vi "Write.vi"(6 "high priority? (F)":bool, 8 "abort (F)":bool, 9 "last element? (F)":bool, 10 "element":T2, 11 "element valid? (T)":bool=TRUE) -> (0 "done?":bool, 2 "channel":T1)   [LabVIEW 2020, in "Event Messenger Priority.lvlib"]
doc: "<p>Writes a value to an Event Messenger <a href=\"nihelplauncher://docs/csh?context=lvcore_lvconcepts_channel_wires_intro\">channel</a> so that the value can be read by one or more <a href=\"nihelplauncher://docs/csh?context=lvcore_glang_event_structure\">Event structures</a>. This endpoint waits if the channel is full.</p>"
uses:
  Event Messenger Priority.lvlib
  <vilib>/event_ctls.llb/usereventprio.ctl
  ChannelOp.ctl
  ))Channel.ctl
  Element.ctl
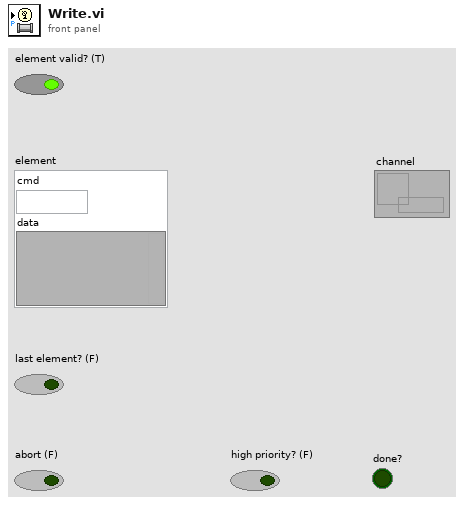
[diagram p1: front panel]
types:
  T1 = typedef "Event Messenger Priority.lvlib/))Channel.ctl" = refnum<queue>
  T2 = typedef "Event Messenger Priority.lvlib/Element.ctl" = cluster{"cmd":string, "data":variant}
  T3 = typedef "usereventprio.ctl" = enum32{"high priority", "normal priority"}
  T4 = typedef "Event Messenger Priority.lvlib/ChannelOp.ctl" = enum16{"init", "write", "register", "replicate", "probe"}
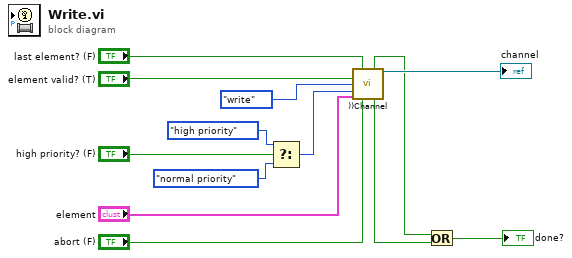
[diagram p0: block diagram]
diagram:
  n1 = Select(t=usereventprio."high priority" ("event priority (normal)"), s="high priority? (F)", f=usereventprio."normal priority" ("event priority (normal)")) -> (s? t:f=w1:T3)
  n2 = call "))Channel.vi"("last element in"="last element? (F)", "valid"="element valid? (T)", "channelOp"=ChannelOp."write", "event priority (norm)"=w1, "element in"="element", "abort in"="abort (F)") -> ("last element out"=w5:bool, "channel out"=→"channel":T1, "aborted?"=w4:bool)  [unwired: 5 in, 2 out]
  n3 = Or(x=w5, y=w4) -> (x .or. y?=→"done?":bool)
